vi "load_array_of_profiles_xml.vi"(8 "error in":errorcluster, 11 "node in":refnum<k20>) -> (0 "error out":errorcluster, 2 "Array of DDS Profiles (8)":T1=[{"Single Tone"={"Frequency [MHz]"=0.0, "Amplitude [dBm]"=0.0, "Phase Offset [rad]"=0.0}, "RAM Mode "=enum."Direct Switch", "Zero-crossing"=FALSE, "No Dwell High"=FALSE, "Function/Static"=FALSE, "RAM Function Settings"=[], "RAM Static Array"=[], "Description"="", "Time Step (us)"=0.0}] {"Time Step (us)" min=0.0 max=262.14 step=0.004 format="%8.3g"}, 3 "node":refnum<k20>)   [LabVIEW 2015, in "DDS.lvclass"]
doc: "Load DDS profile from xml. Expected format:\n\n<profile>\n<SingleTone.Frequency units=\"MHz\">%s</SingleTone.Frequency>\n<SingleTone.Amplitude units=\"dBm\">%s</SingleTone.Amplitude>\n<SingleTone.Phase units=\"rad\">%s</SingleTone.Phase>\n<RAMMode>%u</RAMMode>\n<ZeroCrossing>%b</ZeroCrossing>\n<NoDwellHigh>%b</NoDwellHigh>\n<FunctionOrStatic>%b</FunctionOrStatic>\n<RAMFunctionSettings>%s</RAMFunctionSettings>\n<RAMStaticArray>%s</RAMStaticArray>\n</profile>\n\nMTL 2012 Dec 31"
uses:
  DDS.lvclass
  DDS Library/Controls/DDS Profile Array.ctl
  DDS Library/Controls/DDS Profile.ctl
  DDS Library/Controls/DDS RAM Mode.ctl
  DDS Library/Controls/DDS RAM Timestep.ctl
  <vilib>/xml/Close Reference(Node).vi
  DDS Library/DDS.lvlib
  <resource>/objmgr/DOMUserDefRef.rc
  <vilib>/xml/NI_XML.lvlib
panel:
  # "f/f/A"
  # "Mag"
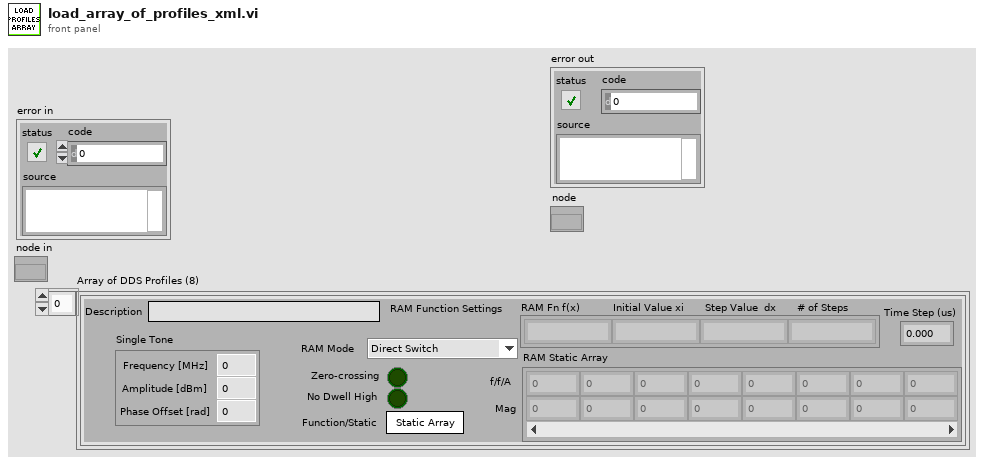
[diagram p1: front panel]
types:
  T1 = typedef "DDS.lvlib/DDS Profile Array.ctl" = T2[]
  T2 = typedef "DDS.lvlib/DDS Profile.ctl" = cluster{"Single Tone":cluster{"Frequency [MHz]":dbl, "Amplitude [dBm]":dbl, "Phase Offset [rad]":dbl}, "RAM Mode ":T3, "Zero-crossing":bool, "No Dwell High":bool, "Function/Static":bool, "RAM Function Settings":string[], "RAM Static Array":dbl[][], "Description":string, "Time Step (us)":T4}
  T3 = typedef "DDS.lvlib/DDS RAM mode.ctl" = enum16{"Direct Switch", "Ramp Up", "Bidirectional Ramp", "Continuous Bidirectional Ramp", "Continuous Recirculate", "Direct Switch 2", "Direct Switch 3", "Direct Switch 4"}
  T4 = typedef "DDS.lvlib/DDS RAM Timestep.ctl" = dbl
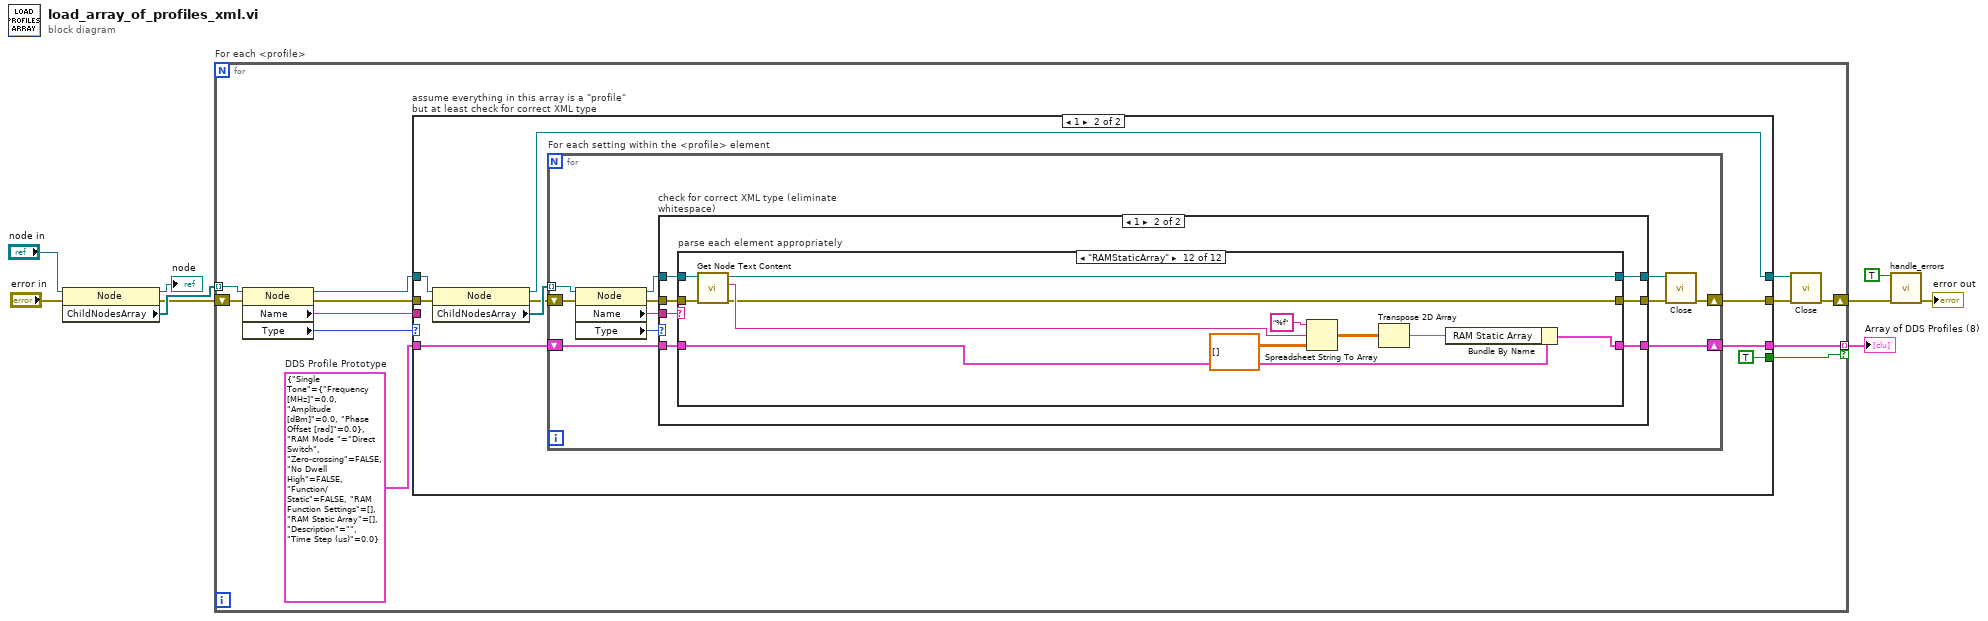
[diagram p0: block diagram]
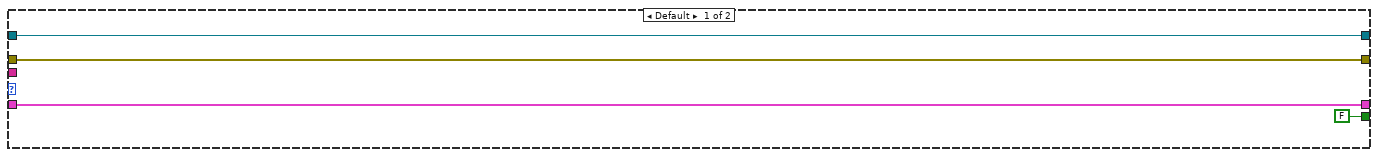
[diagram p2: hidden frame]
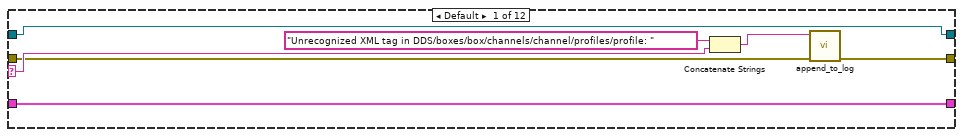
[diagram p4: hidden frame]
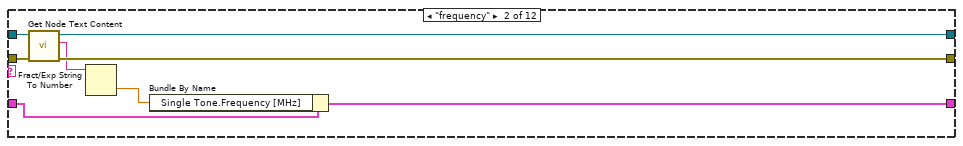
[diagram p5: hidden frame]
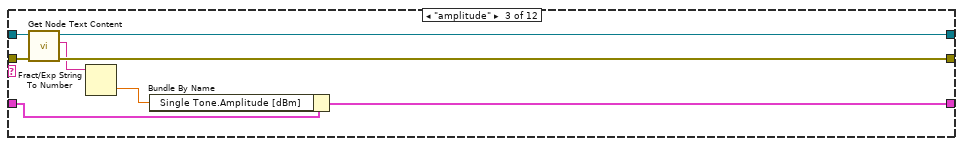
[diagram p6: hidden frame]
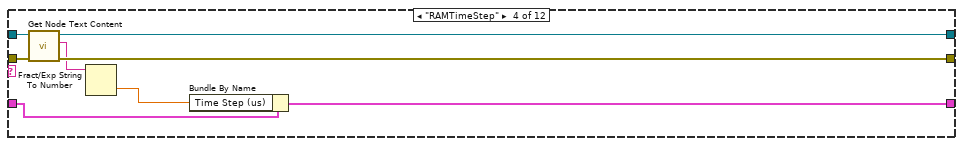
[diagram p7: hidden frame]
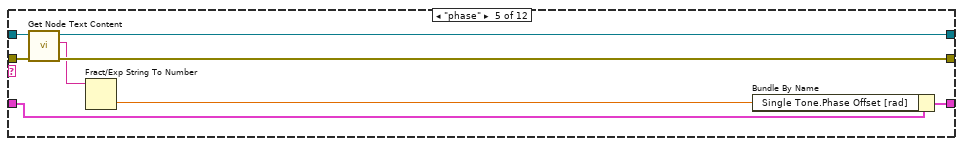
[diagram p8: hidden frame]
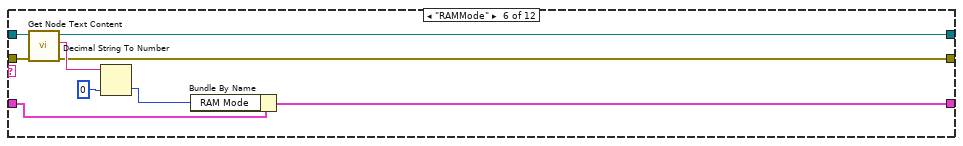
[diagram p9: hidden frame]
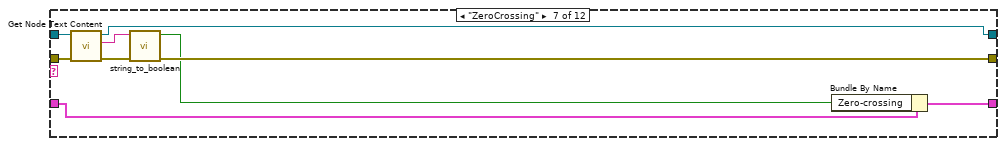
[diagram p10: hidden frame]
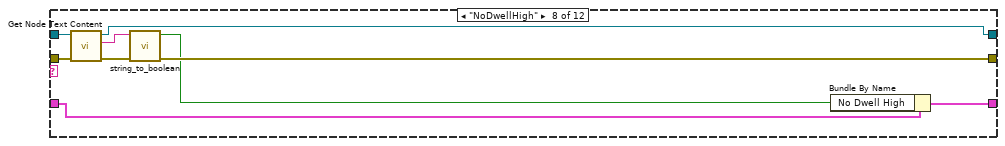
[diagram p11: hidden frame]
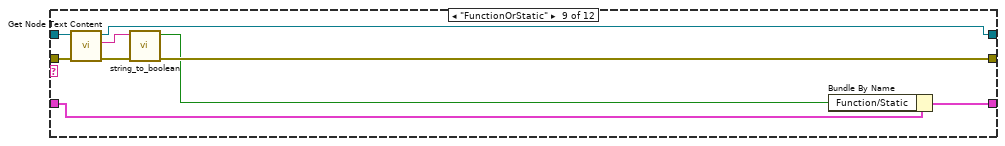
[diagram p12: hidden frame]
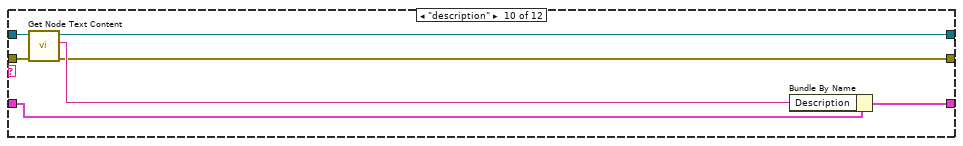
[diagram p13: hidden frame]
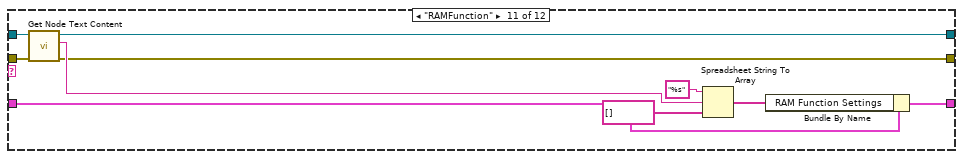
[diagram p14: hidden frame]
diagram:
  n1 = property class="Node"(reference="node in", error in="error in") -> (reference out=→"node":refnum<k20>, error out=w4:errorcluster, "ChildNodesArray"=w6:refnum<k20>[])
  n2 = for "For each <profile>" {
    tunnel: w6 -> [w15] mode=indexing
    shift-right: [w19] -> w3
    shift-left: w4 -> [w17]
    tunnel: [w21] -> w9 mode=indexing if=w10
    w12 = T2 {"Single Tone"={"Frequency [MHz]"=0.0, "Amplitude [dBm]"=0.0, "Phase Offset [rad]"=0.0}, "RAM Mode "=enum."Direct Switch", "Zero-crossing"=FALSE, "No Dwell High"=FALSE, "Function/Static"=FALSE, "RAM Function Settings"=[], "RAM Static Array"=[], "Description"="", "Time Step (us)"=0.0}  # DDS Profile Prototype
    n3 = property class="Node"(reference=w15, error in=w17) -> (reference out=w14:refnum<k20>, error out=w16:errorcluster, "Name"=w11:string, "Type"=w13:i32)
    n4 = case "assume everything in this array is a \"profile\" but at least check for correct XML type" shown="1" w13 {
      tunnel: [w22 w34] -> w21
      tunnel: [w25 w33] -> w20
      tunnel: w14 -> [w24 w32]
      tunnel: [w24 w31] -> w18
      tunnel: w16 -> [w25 w30]
      tunnel: w12 -> [w22 w29]
      tunnel: w11 -> [_ _]
      tunnel: [FALSE TRUE] -> w10
      frame Default {
      }
      frame 1 {
        n5 = property class="Node"(reference=w32, error in=w30) -> (reference out=w31:refnum<k20>, error out=w26:errorcluster, "ChildNodesArray"=w27:refnum<k20>[])
        n6 = for "For each setting within the <profile> element" {
          tunnel: w27 -> [w45] mode=indexing
          shift-right: [w40] -> w33
          shift-left: w26 -> [w43]
          shift-right: [w38] -> w34
          shift-left: w29 -> [w39]
          n7 = property class="Node"(reference=w45, error in=w43) -> (reference out=w37:refnum<k20>, error out=w42:errorcluster, "Name"=w44:string, "Type"=w35:i32)
          n8 = case "check for correct XML type (eliminate whitespace)" shown="1" w35 {
            tunnel: w44 -> [_ w55]
            tunnel: w42 -> [w47 w54]
            tunnel: [w47 w53] -> w41
            tunnel: w39 -> [w48 w52]
            tunnel: [w48 w51] -> w38
            tunnel: w37 -> [w46 w50]
            tunnel: [w46 w49] -> w36
            frame Default {
            }
            frame 1 {
              n9 = case "parse each element appropriately" shown="\"RAMStaticArray\"" w55 {
                selector: w55 -> [w58 _ _ _ _ _ _ _ _ _ _ _]
                tunnel: w54 -> [w57 w68 w76 w84 w90 w98 w109 w118 w128 w135 w143 w157]
                tunnel: [w56 w67 w75 w83 w89 w97 w106 w116 w123 w131 w140 w151] -> w53
                tunnel: w52 -> [w62 w66 w78 w86 w94 w103 w112 w113 w126 w133 w147 w156]
                tunnel: [w62 w65 w73 w81 w93 w102 w111 w119 w130 w137 w146 w155] -> w51
                tunnel: w50 -> [w61 w70 w77 w85 w92 w96 w110 w121 w129 w136 w145 w158]
                tunnel: [w61 w69 w74 w82 w91 w95 w108 w120 w127 w134 w144 w154] -> w49
                frame Default {
                  n10 = Concatenate Strings("Unrecognized XML tag in DDS/boxes/box/channels/channel/profiles/profile: " ("string"), w58) -> (w59:string)
                  n11 = call "append_to_log.vi"("error in"=w57, "string"=w59) -> ("error out"=w56:errorcluster)  [unwired: 9 in]
                }
                frame "frequency" {
                  n12 = call <vilib>:"Get Node Text Content.vi"("error in (no error)"=w68, "node in"=w70) -> ("error out"=w67:errorcluster, "node text"=w64:string, "node out"=w69:refnum<k20>)  [unwired: 7 in]
                  n13 = Fract/Exp String To Number(string=w64) -> (number=w63:dbl)  [unwired: 3 in, 1 out]
                  n14 = Bundle By Name(cluster=w66, "Single Tone.Frequency [MHz]"=w63) -> (w65:T2)
                }
                frame "amplitude" {
                  n15 = call <vilib>:"Get Node Text Content.vi"("error in (no error)"=w76, "node in"=w77) -> ("error out"=w75:errorcluster, "node text"=w72:string, "node out"=w74:refnum<k20>)  [unwired: 7 in]
                  n16 = Fract/Exp String To Number(string=w72) -> (number=w71:dbl)  [unwired: 3 in, 1 out]
                  n17 = Bundle By Name(cluster=w78, "Single Tone.Amplitude [dBm]"=w71) -> (w73:T2)
                }
                frame "RAMTimeStep" {
                  n18 = call <vilib>:"Get Node Text Content.vi"("error in (no error)"=w84, "node in"=w85) -> ("error out"=w83:errorcluster, "node text"=w80:string, "node out"=w82:refnum<k20>)  [unwired: 7 in]
                  n19 = Fract/Exp String To Number(string=w80) -> (number=w79:dbl)  [unwired: 3 in, 1 out]
                  n20 = Bundle By Name(cluster=w86, "Time Step (us)"=w79) -> (w81:T2)
                }
                frame "phase" {
                  n21 = call <vilib>:"Get Node Text Content.vi"("error in (no error)"=w90, "node in"=w92) -> ("error out"=w89:errorcluster, "node text"=w88:string, "node out"=w91:refnum<k20>)  [unwired: 7 in]
                  n22 = Fract/Exp String To Number(string=w88) -> (number=w87:dbl)  [unwired: 3 in, 1 out]
                  n23 = Bundle By Name(cluster=w94, "Single Tone.Phase Offset [rad]"=w87) -> (w93:T2)
                }
                frame "RAMMode" {
                  n24 = call <vilib>:"Get Node Text Content.vi"("error in (no error)"=w98, "node in"=w96) -> ("error out"=w97:errorcluster, "node text"=w101:string, "node out"=w95:refnum<k20>)  [unwired: 7 in]
                  n25 = Decimal String To Number(string=w101, default (0L)=u16 0 ("default (0 I32)")) -> (number=w99:u16)  [unwired: 1 in, 1 out]
                  n26 = Bundle By Name(cluster=w103, "RAM Mode"=w99) -> (w102:T2)
                }
                frame "ZeroCrossing" {
                  n27 = call <vilib>:"Get Node Text Content.vi"("error in (no error)"=w109, "node in"=w110) -> ("error out"=w105:errorcluster, "node text"=w107:string, "node out"=w108:refnum<k20>)  [unwired: 7 in]
                  n28 = call "string_to_boolean.vi"("error in"=w105, "string"=w107) -> ("error out"=w106:errorcluster, "boolean"=w104:bool)  [unwired: 8 in]
                  n29 = Bundle By Name(cluster=w112, "Zero-crossing"=w104) -> (w111:T2)
                }
                frame "NoDwellHigh" {
                  n30 = call <vilib>:"Get Node Text Content.vi"("error in (no error)"=w118, "node in"=w121) -> ("error out"=w115:errorcluster, "node text"=w117:string, "node out"=w120:refnum<k20>)  [unwired: 7 in]
                  n31 = call "string_to_boolean.vi"("error in"=w115, "string"=w117) -> ("error out"=w116:errorcluster, "boolean"=w114:bool)  [unwired: 8 in]
                  n32 = Bundle By Name(cluster=w113, "No Dwell High"=w114) -> (w119:T2)
                }
                frame "FunctionOrStatic" {
                  n33 = call <vilib>:"Get Node Text Content.vi"("error in (no error)"=w128, "node in"=w129) -> ("error out"=w124:errorcluster, "node text"=w125:string, "node out"=w127:refnum<k20>)  [unwired: 7 in]
                  n34 = call "string_to_boolean.vi"("error in"=w124, "string"=w125) -> ("error out"=w123:errorcluster, "boolean"=w122:bool)  [unwired: 8 in]
                  n35 = Bundle By Name(cluster=w126, "Function/Static"=w122) -> (w130:T2)
                }
                frame "description" {
                  n36 = call <vilib>:"Get Node Text Content.vi"("error in (no error)"=w135, "node in"=w136) -> ("error out"=w131:errorcluster, "node text"=w132:string, "node out"=w134:refnum<k20>)  [unwired: 7 in]
                  n37 = Bundle By Name(cluster=w133, "Description"=w132) -> (w137:T2)
                }
                frame "RAMFunction" {
                  n38 = call <vilib>:"Get Node Text Content.vi"("error in (no error)"=w143, "node in"=w145) -> ("error out"=w140:errorcluster, "node text"=w142:string, "node out"=w144:refnum<k20>)  [unwired: 7 in]
                  n39 = Spreadsheet String To Array(format string="%s", spreadsheet string=w142, array type (2D Dbl)=string[] []) -> (array=w138:string[])  [unwired: 1 in]
                  n40 = Bundle By Name(cluster=w147, "RAM Function Settings"=w138) -> (w146:T2)
                }
                frame "RAMStaticArray" {
                  n41 = call <vilib>:"Get Node Text Content.vi"("error in (no error)"=w157, "node in"=w158) -> ("error out"=w151:errorcluster, "node text"=w153:string, "node out"=w154:refnum<k20>)  [unwired: 7 in]
                  n42 = Spreadsheet String To Array(format string="%f", spreadsheet string=w153, array type (2D Dbl)=dbl[][] []) -> (array=w149:dbl[][])  [unwired: 1 in]
                  n43 = Transpose 2D Array(2D array=w149) -> (transposed array=w148:dbl[][])
                  n44 = Bundle By Name(cluster=w156, "RAM Static Array"=w148) -> (w155:T2)
                }
              }
            }
          }
          n45 = call-poly <vilib>:"Close.vi"("error in (no error)"=w41, "node"=w36) -> ("error out"=w40:errorcluster)  [unwired: 7 in]
        }
      }
    }
    n46 = call-poly <vilib>:"Close.vi"("error in (no error)"=w20, "node"=w18) -> ("error out"=w19:errorcluster)  [unwired: 7 in]
  }
  "Array of DDS Profiles (8)" <- w9
  n47 = call "handle_errors.vi"("Exit Operation"=TRUE, "error in (no error)"=w3) -> ("error out"=→"error out":errorcluster)  [unwired: 13 in]
